vi "Move Stage.vi"(8 "error in (no error)":errorcluster, 11 "Ti2 in":refnum<class "Ti2.lvclass">) -> (0 "error out":errorcluster, 3 "Ti2 out":refnum<class "Ti2.lvclass">)   [LabVIEW 2018, in "Ti2.lvlib" / "Ti2.lvclass"]
uses:
  Ti2.lvclass
  Stage Axis.ctl
  ti2lv/ti2lv.lvlib
  Ti2.lvlib
panel:
  in  "Axis":T1
  in  "Relative distance (um)":dbl
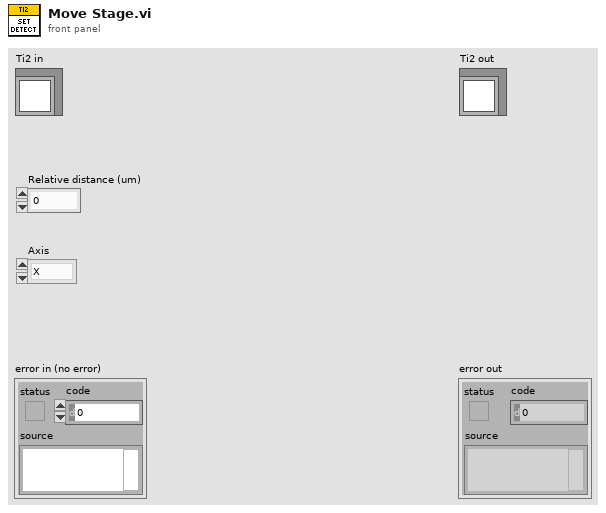
[diagram p1: front panel]
types:
  T1 = typedef "Ti2.lvlib/Stage Axis.ctl" = enum16{"X", "Y", "Z"}
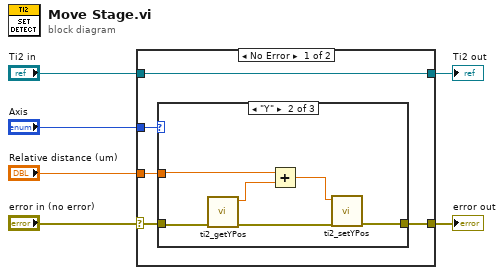
[diagram p0: block diagram]
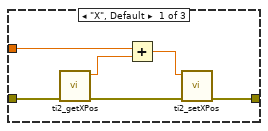
[diagram p2: hidden frame]
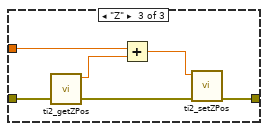
[diagram p3: hidden frame]
diagram:
  n1 = case shown="No Error" "error in (no error)" {
    selector: "error in (no error)" -> [w10 w31]
    tunnel: [w9 w31] -> w5
    tunnel: [w11 w30] -> w3
    tunnel: "Ti2 in" -> [w11 w30]
    tunnel: "Relative distance (um)" -> [w8 _]
    tunnel: "Axis" -> [w7 _]
    frame No Error {
      n2 = case shown="\"Y\"" w7 {
        tunnel: w10 -> [w13 w19 w25]
        tunnel: [w12 w20 w24] -> w9
        tunnel: w8 -> [w14 w18 w26]
        frame "X", Default {
          n3 = call "ti2_getXPos.vi"("error in (no error)"=w13) -> ("error out"=w17:errorcluster, "x Position (um)"=w15:dbl)  [unwired: 9 in]
          n4 = Add(x=w14, y=w15) -> (x+y=w16:dbl)
          n5 = call "ti2_setXPos.vi"("error in (no error)"=w17, "x Position (um)"=w16) -> ("error out"=w12:errorcluster)  [unwired: 9 in]
        }
        frame "Y" {
          n6 = call "ti2_getYPos.vi"("error in (no error)"=w19) -> ("error out"=w21:errorcluster, "y Position (um)"=w23:dbl)  [unwired: 9 in]
          n7 = Add(x=w18, y=w23) -> (x+y=w22:dbl)
          n8 = call "ti2_setYPos.vi"("error in (no error)"=w21, "y Position (um)"=w22) -> ("error out"=w20:errorcluster)  [unwired: 9 in]
        }
        frame "Z" {
          n9 = call "ti2_getZPos.vi"("error in (no error)"=w25) -> ("error out"=w29:errorcluster, "z Position (um)"=w27:dbl)  [unwired: 9 in]
          n10 = Add(x=w26, y=w27) -> (x+y=w28:dbl)
          n11 = call "ti2_setZPos.vi"("error in (no error)"=w29, "z Position (um)"=w28) -> ("error out"=w24:errorcluster)  [unwired: 9 in]
        }
      }
    }
    frame Error {
    }
  }
  "error out" <- w5
  "Ti2 out" <- w3
